vi "Condition ROI data.vi"(8 "error in (no error)":errorcluster, 10 "Data for ticked ROI":T1=[{"Plot.Plot Name"="1: Point", "Data"={"X-Axis values"=array[43860 elements], "Y-Axis values (s)"=array[43860 elements]}, "Timeline data"={"X-Axis values"=[], "Y-Axis values (s)"=[]}, "Type"=enum."Mini-scan", "Points per cycle"=1, "ROI number"=0}], 11 "Data for ticked Groups":T1) -> (0 "error out":errorcluster, 3 "Data reference":refnum<data-value>)   [LabVIEW 2017]
uses:
  xcontrol/Interface VIs/Interface typedefs/Interface-Data array.ctl
  xcontrol/Interface VIs/Interface typedefs/Interface-Data format definition.ctl
  xcontrol/Typedefs/Xctl-XY data type definition.ctl
  xcontrol/Typedefs/Xctrl-ROI type enum.ctl
  xcontrol/XGrapher.xctl
panel:
  out "Averaged":bool
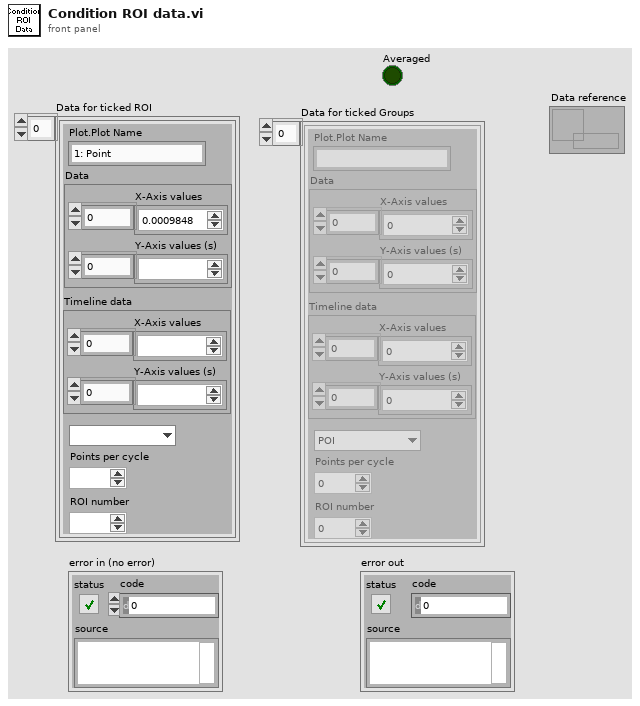
[diagram p1: front panel]
types:
  T1 = typedef "Interface-Data array.ctl" = T2[]
  T2 = typedef "Interface-Data format definition.ctl" = cluster{"Plot.Plot Name":string, "Data":T3, "Timeline data":T3, "Type":T4, "Points per cycle":u16, "ROI number":u16}
  T3 = typedef "XGrapher.xctl/Xctl-XY data type definition.ctl" = cluster{"X-Axis values":sgl[], "Y-Axis values (s)":sgl[]}
  T4 = typedef "Xctrl-ROI type enum.ctl" = enum16{"POI", "Mini-scan", "Group"}
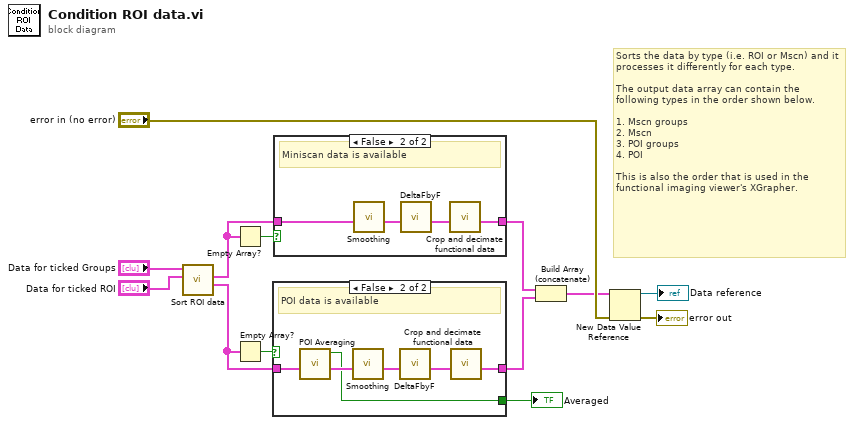
[diagram p0: block diagram]
diagram:
  # "Sorts the data by type (i.e. ROI or Mscn) and it processes it differently for each type.\n\nThe output data array can contain the following types in the order shown below.\n\n1. Mscn groups\n2. Mscn\n3. POI groups\n4. POI\n\nThis is also the order that is used in the functional imaging viewer's XGrapher."
  n1 = call "Sort ROI data.vi"("Data for ticked ROI"="Data for ticked ROI", "Data for ticked Groups"="Data for ticked Groups") -> ("POI  and POI groups raw data"=w6:T1, "Miniscans and Mscn groups raw data"=w5:T1)  [unwired: 8 in]
  n2 = Empty Array?(array=w5) -> (empty?=w11:bool)
  n3 = Empty Array?(array=w6) -> (empty?=w10:bool)
  n4 = case shown="False" w10 {
    tunnel: w6 -> [w14 w18]
    tunnel: [w14 w15] -> w13
    tunnel: [_ w17] -> w1
    frame True {
      # "No POI data available"
    }
    frame False {
      # "POI data is available"
      n5 = call "POI Averaging.vi"("Data in"=w18) -> ("Data out"=w19:T1, "Averaged"=w17:bool)  [unwired: 9 in]
      n6 = call "Smoothing.vi"("Data in"=w19) -> ("Data out"=w20:T1)  [unwired: 10 in]
      n7 = call "DeltaFbyF.vi"("Data in"=w20) -> ("Data out"=w16:T1)  [unwired: 10 in]
      n8 = call "Crop and decimate functional data.vi"("Data in"=w16) -> ("Data out"=w15:T1)  [unwired: 10 in]
    }
  }
  "Averaged" <- w1
  n9 = case shown="False" w11 {
    tunnel: w5 -> [w21 w24]
    tunnel: [w21 w22] -> w12
    frame True {
      # "No miniscan data available"
    }
    frame False {
      # "Miniscan data is available"
      n10 = call "Smoothing.vi"("Data in"=w24) -> ("Data out"=w25:T1)  [unwired: 10 in]
      n11 = call "DeltaFbyF.vi"("Data in"=w25) -> ("Data out"=w23:T1)  [unwired: 10 in]
      n12 = call "Crop and decimate functional data.vi"("Data in"=w23) -> ("Data out"=w22:T1)  [unwired: 10 in]
    }
  }
  n13 = Build Array (concatenate)(w12, w13) -> (w4:T1)
  n14 = New Data Value Reference(data value=w4, error in="error in (no error)") -> (data value reference=→"Data reference":refnum<data-value>, error out=→"error out":errorcluster)
